vi "populate Tree from Data.vi"(6 "error in (no error)":errorcluster, 8 "Data":T1={"Report.lvclass"=refnum, "Norm"="", "last State"=enum."Initialize", "Norm ID"=0, "parameter"=[], "EMTestCWS500N.lvclass"=refnum, "CEG4500.lvclass"=refnum, "Tektronix RSA5106A.lvclass"=refnum, "erfolgreich"=FALSE, "log"="", "Kommentar"="", "Device Enum"=enum."emTestCWS500N", "Test Enum"=enum."HF-Felder", "debug"=FALSE, "tab"=enum."Hauptmenü", "ESD Pistol.lvclass"=refnum, "SubPnl Refnum"=refnum, "TabCtl Refnum"=refnum, "ButtonsEinblenden?"=FALSE}, 9 "reference":refnum<vi>) -> (0 "error out":errorcluster)   [LabVIEW 2013, in "TreeRepresentation.lvlib"]
doc: "Prüfdaten in die Baumstruktur unter dem Prüfdatenreiter eintragen"
uses:
  lib/TreeRepresentation.lvlib
  Main/controls/Data.ctl
  classes/Datastructure/Report/Report.lvclass
  classes/Devices/emTestCWS500N/EMTestCWS500N.lvclass
  classes/Devices/CEG4500/CEG4500.lvclass
  classes/Devices/Tektronix RSA5106A/Tektronix RSA5106A.lvclass
  ESD Pistol.lvclass
  Main/controls/State.ctl
  classes/Devices/DeviceInterface/Devices.ctl
  classes/Tests/TestInterface/Tests.ctl
  Tabs.ctl
  classes/Datastructure/Norm/Norm.lvclass
  classes/Datastructure/Setup/Setup.lvclass
  classes/Datastructure/Image/img.lvclass
  classes/Datastructure/Device/Device.lvclass
  classes/Datastructure/Test/Test.lvclass
panel:
  out "reference 2":refnum<vi>
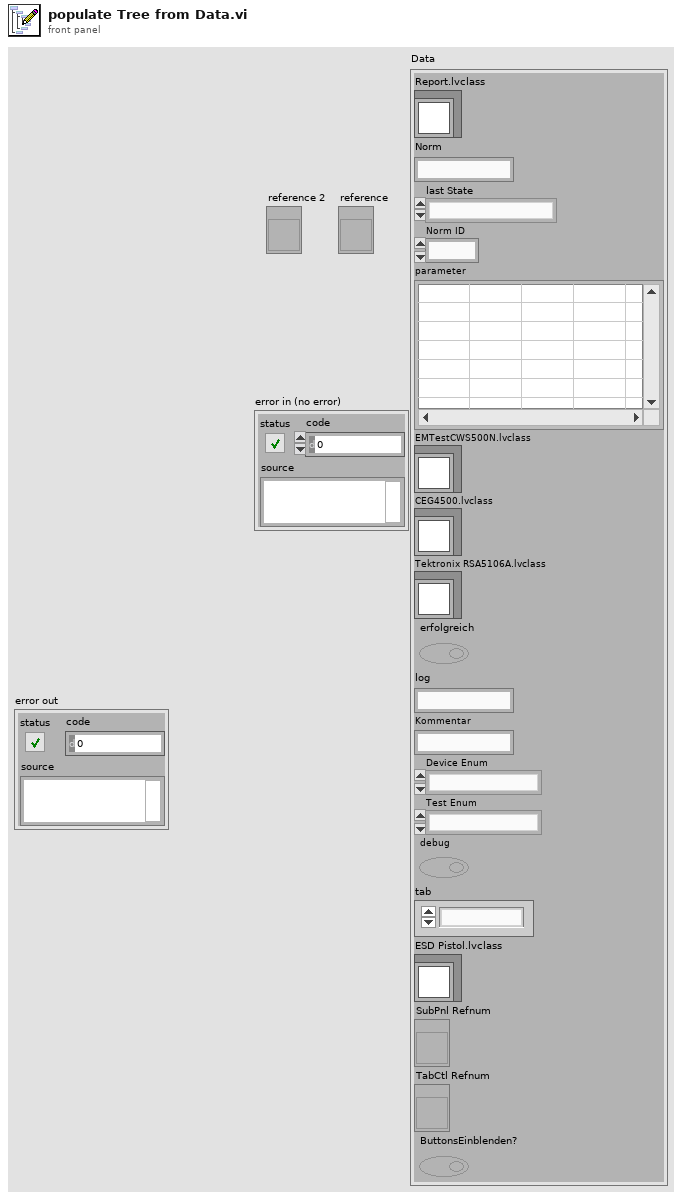
[diagram p1: front panel]
types:
  T1 = typedef "Data.ctl" = cluster{"Report.lvclass":refnum<class "Report.lvclass">, "Norm":string, "last State":T2, "Norm ID":i32, "parameter":string[][], "EMTestCWS500N.lvclass":refnum<class "EMTestCWS500N.lvclass">, "CEG4500.lvclass":refnum<class "CEG4500.lvclass">, "Tektronix RSA5106A.lvclass":refnum<class "Tektronix RSA5106A.lvclass">, "erfolgreich":bool, "log":string, "Kommentar":string, "Device Enum":T3, "Test Enum":T4, "debug":bool, "tab":T5, "ESD Pistol.lvclass":refnum<class "ESD Pistol.lvclass">, "SubPnl Refnum":refnum<vi>, "TabCtl Refnum":refnum<vi>, "ButtonsEinblenden?":bool}
  T2 = typedef "State.ctl" = enum16{"create Pdf", "load Report", "save Report", "do Test", "CDN Kalibrierung", "enter Report Parameters", "new Test", "Protokoll", "read Tree", "update Tree", "Fehler", "Initialize", "Wait for Event", "Exit"}
  T3 = typedef "Devices.ctl" = enum16{"unbekannt", "ESD Pistol", "Tektronix RSA5106A", "emTestCWS500N", "CEG-4500"}
  T4 = typedef "Tests.ctl" = enum16{"unbekannt", "Störaussendung", "Burst", "ESD", "Surge", "Spannungseinbruch", "HF-Felder"}
  T5 = typedef "Tabs.ctl" = enum32{"Hauptmenü", "Prüfbericht", "Einstellungen"}
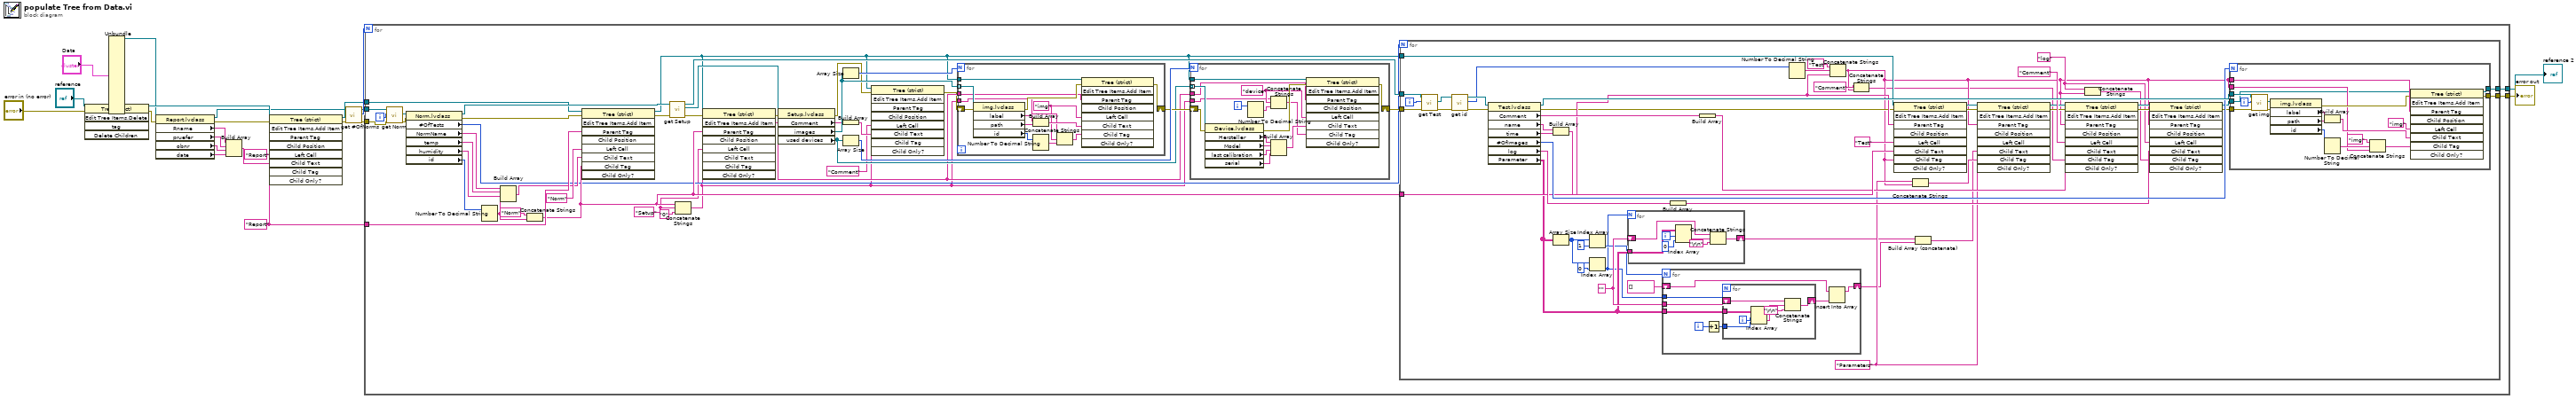
[diagram p0: block diagram]
diagram:
  w21 = "Report" ("Child Tag")
  n1 = invoke on="Invoke Node" class="Tree (strict)" method="Edit Tree Items.Delete"(reference="reference", error in="error in (no error)") -> (reference out=w11:refnum<vi>, error out=w5:errorcluster)  [unwired: 3 in, 3 out]
  n2 = Unbundle("Data") -> ("Report.lvclass"=w8:refnum<class "Report.lvclass">)  [unwired: 18 out]
  n3 = property class="Report.lvclass"(reference=w8, error in=w5) -> (reference out=w7:refnum<class "Report.lvclass">, error out=w6:errorcluster, "Rname"=w4:string, "pruefer"=w3:string, "obnr"=w2:string, "date"=w1:string)
  n4 = Build Array(w4, w3, w2, w1) -> (w19:string[])
  n5 = invoke on="Invoke Node" class="Tree (strict)" method="Edit Tree Items.Add Item"(reference=w11, error in=w6, "Left Cell"="Report" ("Left Cell String"), "Child Text"=w19, "Child Tag"=w21) -> (reference out=w10:refnum<vi>, error out=w14:errorcluster)  [unwired: 4 in, 7 out]
  n6 = call-dynamic "get #OfNorms.vi"("error in (no error)"=w14, "Report (Eingang)"=w7) -> ("error out"=w13:errorcluster, "#OfTests"=w18:u32, "Report (Ausgang)"=w17:refnum<class "Report.lvclass">)  [unwired: 7 in]
  n7 = for {
    N: w18 -> [_]
    tunnel: w13 -> [w60]
    tunnel: w21 -> [w63]
    tunnel: w17 -> [w61]
    tunnel: [w58] -> w16
    tunnel: w10 -> [w49]
    tunnel: [w48] -> w9
    i -> [w52]
    w25 = "Setup" ("Linker Zellen-String")
    n8 = call-dynamic "get Norm.vi"("error in (no error)"=w60, "index"=w52, "Report (Eingang)"=w61) -> ("error out"=w57:errorcluster, "Norm"=w56:refnum<class "Norm.lvclass">)  [unwired: 6 in, 1 out]
    n9 = property class="Norm.lvclass"(reference=w56, error in=w57) -> (reference out=w55:refnum<class "Norm.lvclass">, error out=w54:errorcluster, "#OfTests"=w29:u32, "NormName"=w53:string, "temp"=w47:string, "humidity"=w46:string, "id"=w26:i32)
    n10 = Number To Decimal String(number=w26) -> (decimal integer string=w27:string)  [unwired: 1 in]
    n11 = Build Array(w53, w47, w46, w27) -> (w59:string[])
    n12 = Concatenate Strings("Norm" ("Child Tag"), w27) -> (w50:string)
    n13 = invoke on="Invoke Node" class="Tree (strict)" method="Edit Tree Items.Add Item"(reference=w49, error in=w54, "Parent Tag"=w63, "Left Cell"="Norm" ("Left Cell String"), "Child Text"=w59, "Child Tag"=w50) -> (reference out=w28:refnum<vi>, error out=w62:errorcluster)  [unwired: 3 in, 7 out]
    n14 = call-dynamic "get Setup.vi"("error in (no error)"=w62, "Norm (Eingang)"=w55) -> ("error out"=w37:errorcluster, "Setup.lvclass"=w44:refnum<class "Setup.lvclass">, "Norm (Ausgang)"=w45:refnum<class "Norm.lvclass">)  [unwired: 7 in]
    n15 = Concatenate Strings(w50, w25, "0" ("string")) -> (w23:string)
    n16 = invoke on="Invoke Node" class="Tree (strict)" method="Edit Tree Items.Add Item"(reference=w28, error in=w37, "Parent Tag"=w50, "Left Cell"=w25, "Child Tag"=w23) -> (error out=w36:errorcluster, "Edit Tree Items:Add Item"=w35:string)  [unwired: 4 in, 7 out]
    n17 = property class="Setup.lvclass"(reference=w44, error in=w36) -> (error out=w34:errorcluster, "Comment"=w32:string, "images"=w42:refnum<class "img.lvclass">[], "used devices"=w38:refnum<class "Device.lvclass">[])  [unwired: 1 out]
    n18 = Array Size(array=w42) -> (size(s)=w43:i32)
    n19 = Build Array(w32) -> (w31:string[])
    n20 = Array Size(array=w38) -> (size(s)=w41:i32)
    n21 = invoke on="Invoke Node" class="Tree (strict)" method="Edit Tree Items.Add Item"(reference=w28, error in=w34, "Parent Tag"=w23, "Left Cell"="Comment" ("Linker Zellen-String"), "Child Text"=w31) -> (error out=w33:errorcluster)  [unwired: 4 in, 8 out]
    n22 = for {
      N: w43 -> [_]
      tunnel: w42 -> [w185] mode=indexing
      tunnel: w28 -> [w187]
      shift-right: [w186] -> w40
      shift-left: w33 -> [w184]
      tunnel: w23 -> [w179]
      tunnel: w35 -> [w175]
      w178 = "img" ("Linker Zellen-String")
      n23 = property class="img.lvclass"(reference=w185, error in=w184) -> (error out=w183:errorcluster, "label"=w182:string, "path"=w181:string, "id"=w174:i32)  [unwired: 1 out]
      n24 = Build Array(w182, w181) -> (w180:string[])
      n25 = Number To Decimal String(number=w174) -> (decimal integer string=w177:string)  [unwired: 1 in]
      n26 = Concatenate Strings(w179, w178, w177) -> (w176:string)
      n27 = invoke on="Invoke Node" class="Tree (strict)" method="Edit Tree Items.Add Item"(reference=w187, error in=w183, "Parent Tag"=w175, "Left Cell"=w178, "Child Text"=w180, "Child Tag"=w176) -> (error out=w186:errorcluster)  [unwired: 3 in, 8 out]
    }
    n28 = for {
      N: w41 -> [_]
      tunnel: w28 -> [w159]
      shift-right: [w173] -> w39
      shift-left: w40 -> [w171]
      tunnel: w38 -> [w172] mode=indexing
      tunnel: w23 -> [w161]
      tunnel: w35 -> [w160]
      i -> [w165]
      w164 = "device" ("Linker Zellen-String")
      n29 = property class="Device.lvclass"(reference=w172, error in=w171) -> (error out=w170:errorcluster, "Hersteller"=w169:string, "Model"=w168:string, "last calibration"=w167:string, "serial"=w158:string)  [unwired: 1 out]
      n30 = Number To Decimal String(number=w165) -> (decimal integer string=w163:string)  [unwired: 1 in]
      n31 = Concatenate Strings(w161, w164, w163) -> (w162:string)
      n32 = Build Array(w169, w168, w167, w158) -> (w166:string[])
      n33 = invoke on="Invoke Node" class="Tree (strict)" method="Edit Tree Items.Add Item"(reference=w159, error in=w170, "Parent Tag"=w160, "Left Cell"=w164, "Child Text"=w166, "Child Tag"=w162) -> (error out=w173:errorcluster)  [unwired: 3 in, 8 out]
    }
    n34 = for {
      N: w29 -> [_]
      tunnel: [w108] -> w58
      tunnel: [w104] -> w48
      tunnel: w45 -> [w97]
      tunnel: w39 -> [w96]
      tunnel: w50 -> [w95]
      tunnel: w28 -> [w90]
      i -> [w70]
      w82 = ""
      w88 = "Parameters" ("Linker Zellen-String")
      w86 = "log" ("Linker Zellen-String")
      n35 = call-dynamic "get Test.vi"("error in (no error)"=w96, "index"=w70, "Norm (Eingang)"=w97) -> ("error out"=w69:errorcluster, "Test.lvclass"=w68:refnum<class "Test.lvclass">)  [unwired: 6 in, 1 out]
      n36 = call-dynamic "get id.vi"("error in (no error)"=w69, "Test in"=w68) -> ("error out"=w67:errorcluster, "id"=w65:u32, "Test out"=w66:refnum<class "Test.lvclass">)  [unwired: 7 in]
      n37 = property class="Test.lvclass"(reference=w66, error in=w67) -> (reference out=w110:refnum<class "Test.lvclass">, error out=w89:errorcluster, "Comment"=w111:string, "name"=w114:string, "time"=w113:string, "#OfImages"=w109:u32, "log"=w98:string, "Parameter"=w77:string[][])
      n38 = Build Array(w114, w113) -> (w115:string[])
      n39 = Array Size(array=w77) -> (size(s)=w75:i32[])
      n40 = Index Array(array=w75, index=1 ("Index")) -> (element=w72:i32)
      n41 = Index Array(array=w75, index=0 ("Index")) -> (element=w71:i32)
      n42 = for {
        N: w71 -> [_]
        tunnel: w77 -> [w137]
        shift-right: [w138] -> w84
        shift-left: w82 -> [w136]
        i -> [w135]
        n43 = Index Array(array=w137, index (row)=w135, index (col)=0 ("Deaktivierter Index (Spalte)")) -> (element=w132:string)
        n44 = Concatenate Strings(w136, w132, "\r\n") -> (w138:string)
      }
      n45 = for {
        N: w72 -> [_]
        tunnel: w82 -> [w124]
        tunnel: w71 -> [w123]
        tunnel: w77 -> [w122]
        shift-right: [w120] -> w81
        shift-left: string[] [] -> [w119]
        i -> [w117]
        n46 = Increment(x=w117) -> (x+1=w118:i32)
        n47 = for {
          N: w123 -> [_]
          tunnel: w122 -> [w130]
          shift-right: [w131] -> w121
          shift-left: w124 -> [w129]
          tunnel: w118 -> [w127]
          i -> [w126]
          n48 = Index Array(array=w130, index (row)=w126, index (col)=w127) -> (element=w128:string)
          n49 = Concatenate Strings(w129, w128, "\r\n") -> (w131:string)
        }
        n50 = Insert Into Array(array=w119, new element=w121) -> (w120:string[])  [unwired: 1 in]
      }
      n51 = Build Array(w98) -> (w101:string[])
      n52 = Build Array(w111) -> (w112:string[])
      n53 = Number To Decimal String(number=w65) -> (decimal integer string=w106:string)  [unwired: 1 in]
      n54 = Concatenate Strings("Test" ("Child Tag"), w106, w95) -> (w79:string)
      n55 = Concatenate Strings("Comment" ("Child Tag"), w79) -> (w78:string)
      n56 = invoke on="Invoke Node" class="Tree (strict)" method="Edit Tree Items.Add Item"(reference=w90, error in=w89, "Parent Tag"=w95, "Left Cell"="Test" ("Left Cell String"), "Child Text"=w115, "Child Tag"=w79) -> (reference out=w92:refnum<vi>, error out=w91:errorcluster)  [unwired: 3 in, 7 out]
      n57 = Concatenate Strings(w88, w79) -> (w87:string)
      n58 = Build Array (concatenate)(w84, w81) -> (w83:string[])
      n59 = invoke on="Invoke Node" class="Tree (strict)" method="Edit Tree Items.Add Item"(reference=w92, error in=w91, "Parent Tag"=w79, "Left Cell"=w88, "Child Text"=w83, "Child Tag"=w87) -> (reference out=w94:refnum<vi>, error out=w93:errorcluster)  [unwired: 3 in, 7 out]
      n60 = invoke on="Invoke Node" class="Tree (strict)" method="Edit Tree Items.Add Item"(reference=w94, error in=w93, "Parent Tag"=w79, "Left Cell"="Comment" ("Left Cell String"), "Child Text"=w112, "Child Tag"=w78) -> (reference out=w103:refnum<vi>, error out=w102:errorcluster)  [unwired: 3 in, 7 out]
      n61 = Concatenate Strings(w86, w79) -> (w85:string)
      n62 = invoke on="Invoke Node" class="Tree (strict)" method="Edit Tree Items.Add Item"(reference=w103, error in=w102, "Parent Tag"=w79, "Left Cell"=w86, "Child Text"=w101, "Child Tag"=w85) -> (reference out=w100:refnum<vi>, error out=w99:errorcluster)  [unwired: 3 in, 7 out]
      n63 = for {
        N: w109 -> [_]
        tunnel: w99 -> [w157]
        tunnel: w110 -> [w156]
        tunnel: w79 -> [w150]
        tunnel: [w148] -> w108
        tunnel: w79 -> [w143]
        tunnel: w100 -> [w142]
        tunnel: [w141] -> w104
        i -> [w140]
        n64 = call-dynamic "get img.vi"("error in (no error)"=w157, "index"=w140, "Test (Eingang)"=w156) -> ("error out"=w154:errorcluster, "img.lvclass"=w155:refnum<class "img.lvclass">)  [unwired: 6 in, 1 out]
        n65 = property class="img.lvclass"(reference=w155, error in=w154) -> (error out=w149:errorcluster, "label"=w153:string, "path"=w152:string, "id"=w139:i32)  [unwired: 1 out]
        n66 = Build Array(w153, w152) -> (w151:string[])
        n67 = Number To Decimal String(number=w139) -> (decimal integer string=w144:string)  [unwired: 1 in]
        n68 = Concatenate Strings("img" ("Child Tag"), w144, w143) -> (w146:string)
        n69 = invoke on="Invoke Node" class="Tree (strict)" method="Edit Tree Items.Add Item"(reference=w142, error in=w149, "Parent Tag"=w150, "Left Cell"="img" ("Left Cell String"), "Child Text"=w151, "Child Tag"=w146) -> (reference out=w141:refnum<vi>, error out=w148:errorcluster)  [unwired: 3 in, 7 out]
      }
    }
  }
  "error out" <- w16
  "reference 2" <- w9
